vi "Find Table Key-Value Pair.vi"(8 "error in (no error)":errorcluster, 10 "Table Array":string[][](array[string]), 11 "Key Regex":string) -> (0 "error out":errorcluster, 3 "Value":string)   [LabVIEW 2025, in "Test Limits.lvlib"]
uses:
  Test Limits.lvlib
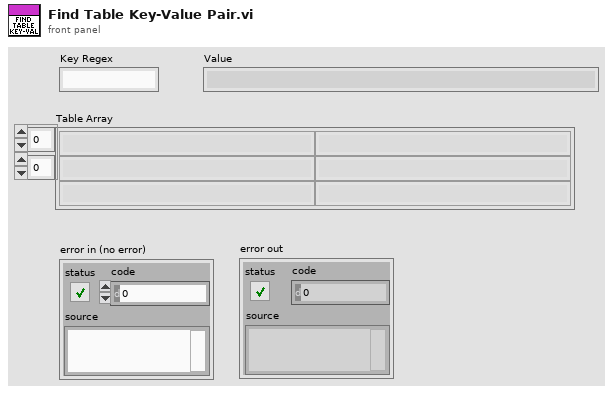
[diagram p1: front panel]
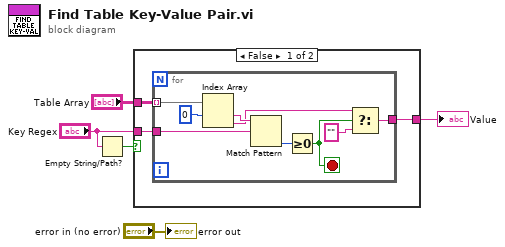
[diagram p0: block diagram]
diagram:
  n1 = Empty String/Path?(string/path="Key Regex") -> (empty?=w4:bool)
  n2 = case shown="False" w4 {
    tunnel: "Table Array" -> [w8 _]
    tunnel: [w7 _] -> w3
    tunnel: "Key Regex" -> [w6 _]
    frame False {
      n3 = for {
        tunnel: w8 -> [w17] mode=indexing
        tunnel: [w10] -> w7
        tunnel: w6 -> [w9]
        stop <- w13 stop-if-true
        n4 = Index Array(array=w17, index #1=0 ("index")) -> (element #1=w15:string, element #2=w12:string)  [unwired: 1 in]
        n5 = Match Pattern(string=w15, regular expression=w9) -> (offset past match=w14:i32)  [unwired: 1 in, 3 out]
        n6 = Greater Or Equal To 0?(x=w14) -> (x >= 0?=w13:bool)
        n7 = Select(t=w12, s=w13, f="") -> (s? t:f=w10:string)
      }
    }
    frame True {
    }
  }
  "Value" <- w3
  "error out" <- "error in (no error)"
